vi "Example VISA GRBL.vi"() -> ()   [LabVIEW 2014]
uses:
  vi.lib/Q-WaveSystems/QwaveSys Raspberry Pi for LabVIEW Home-Education/QwaveSys Raspberry Pi Library.lvlib
panel:
  in  "GRBL Cmd":string[](array[string])=["G10P0L20X0Y0", "G90", "G00X40", "G00Y80", "G00X0Y0", "M30"]
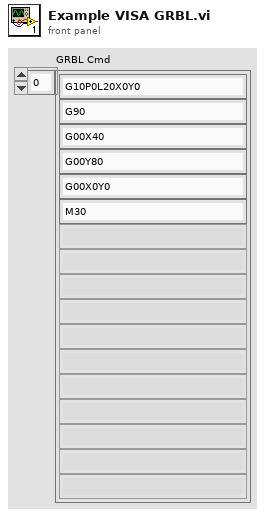
[diagram p1: front panel]
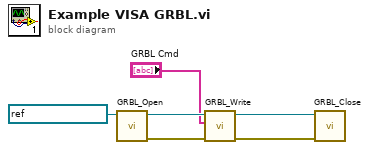
[diagram p0: block diagram]
diagram:
  n1 = call "GRBL_Open.vi"("VISA resource name"=refnum<visa-resource-name> "ASRL1::INSTR") -> ("error out"=w3:errorcluster, "VISA resource name out"=w6:refnum<visa-resource-name>)  [unwired: 9 in]
  n2 = call "GRBL_Write .vi"("error in"=w3, "GRBL Cmd"="GRBL Cmd", "VISA resource name"=w6) -> ("error out"=w2:errorcluster, "VISA resource name out"=w5:refnum<visa-resource-name>)  [unwired: 7 in]
  n3 = call "GRBL_Close.vi"("error in (no error)"=w2, "VISA resource name"=w5) -> ()  [unwired: 10 in]
